vi "GetXMLArrayTags.vi"(2 "ArrayTag":string, 3 "String":string) -> (0 "Array":string[](array[string]), 1 "String w/o tag":string)   [LabVIEW 2010]
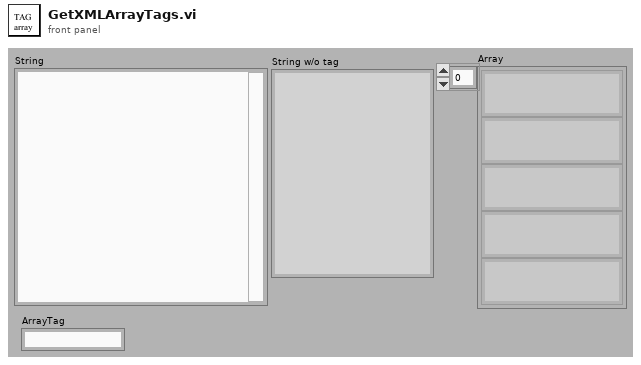
[diagram p1: front panel]
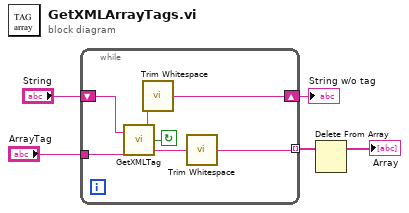
[diagram p0: block diagram]
diagram:
  n1 = while {
    shift-right: [w10] -> w2
    shift-left: "String" -> [w12]
    tunnel: "ArrayTag" -> [w9]
    tunnel: [w7] -> w5 mode=indexing
    stop <- w6 continue-if-true
    n2 = call "GetXMLTag.vi"("Tag"=w9, "String"=w12) -> ("Value"=w8:string, "Exists?"=w6:bool, "String w/o Tag"=w11:string)
    n3 = call <vilib>:"Trim Whitespace.vi"("string"=w11) -> ("trimmed string"=w10:string)  [unwired: 1 in]
    n4 = call <vilib>:"Trim Whitespace.vi"("string"=w8) -> ("trimmed string"=w7:string)  [unwired: 1 in]
  }
  "String w/o tag" <- w2
  n5 = Delete From Array(array=w5) -> (array with subset deleted=→"Array":string[])  [unwired: 2 in, 1 out]
